vi "GUI_HTT_Logger.vi"() -> ()   [LabVIEW 2013]
uses:
  Shared/GUI_Template/GUI_master/tcp_new_data_event.ctl
  Shared/GUI_Template/GUI_master/tcp new data cluster.ctl
panel:
  out "PellicleMeter 10h":cluster{"Y":dbl[], "Y":dbl[]}[](graph)
  out "PellicleMeter":cluster{"Y":dbl[], "Y":dbl[]}[](graph)
  in  "AI_mean.Channel 0::4":dbl caption="Temperature" min=0.0 max=0.0
  in  "GUIdevice 4":string="HTT-PellicleMeter"
  in  "Energy.Channel 1::2":dbl caption="Energy" min=0.0 max=0.0
  in  "Energy.Channel 0::2":dbl min=0.0 max=20.0
  out "Energy 2 10h":cluster{"Y":dbl[], "Y":dbl[]}[](graph)
  out "Temp Gaia 10h":cluster{"Y":dbl[], "Y":dbl[]}[](graph)
  out "Temp Amps 10h":cluster{"Y":dbl[], "Y":dbl[]}[](graph)
  out "Temp Amps":cluster{"Y":dbl[], "Y":dbl[]}[](graph)
  in  "GUIdevice 3":string="HTT-Temp-Amps"
  in  "Temperature::3":dbl caption="Temperature" min=0.0 max=500.0
  in  "Temperature::1":dbl caption="Temperature" min=0.0 max=500.0
  in  "GUIdevice 2":string="HTT-Pulsar"
  in  "Wavelength.Channel1::2":string(combo)="800"
  in  "EnergyRange.Channel1::2":string(combo)="4.00J"
  in  "MeasurementMode.Channel1::2":string(combo)="Energy"
  in  "Wavelength.Channel0::2":string(combo)="800"
  in  "EnergyRange.Channel0::2":string(combo)="4.00J"
  in  "MeasurementMode.Channel0::2":string(combo)="Energy"
  out "tcp data event":T1
  out "error IO 2":errorcluster
  in  "ExternalTrigger.Channel1::2":bool=TRUE caption="Blank Button"
  in  "GUIdevice 1":string="HTT-Temp-Gaia"
  in  "?":bool
  out "Energy 2":cluster{"Y":dbl[], "Y":dbl[]}[](graph)
  out "Temp Gaia":cluster{"Y":dbl[], "Y":dbl[]}[](graph)
  out "Energy 1":cluster{"Y":dbl[], "Y":dbl[]}[](graph)
  out "Energy 1 10h":cluster{"Y":dbl[], "Y":dbl[]}[](graph)
  # "Please re-enter these values after starting the program or restarting the device!"
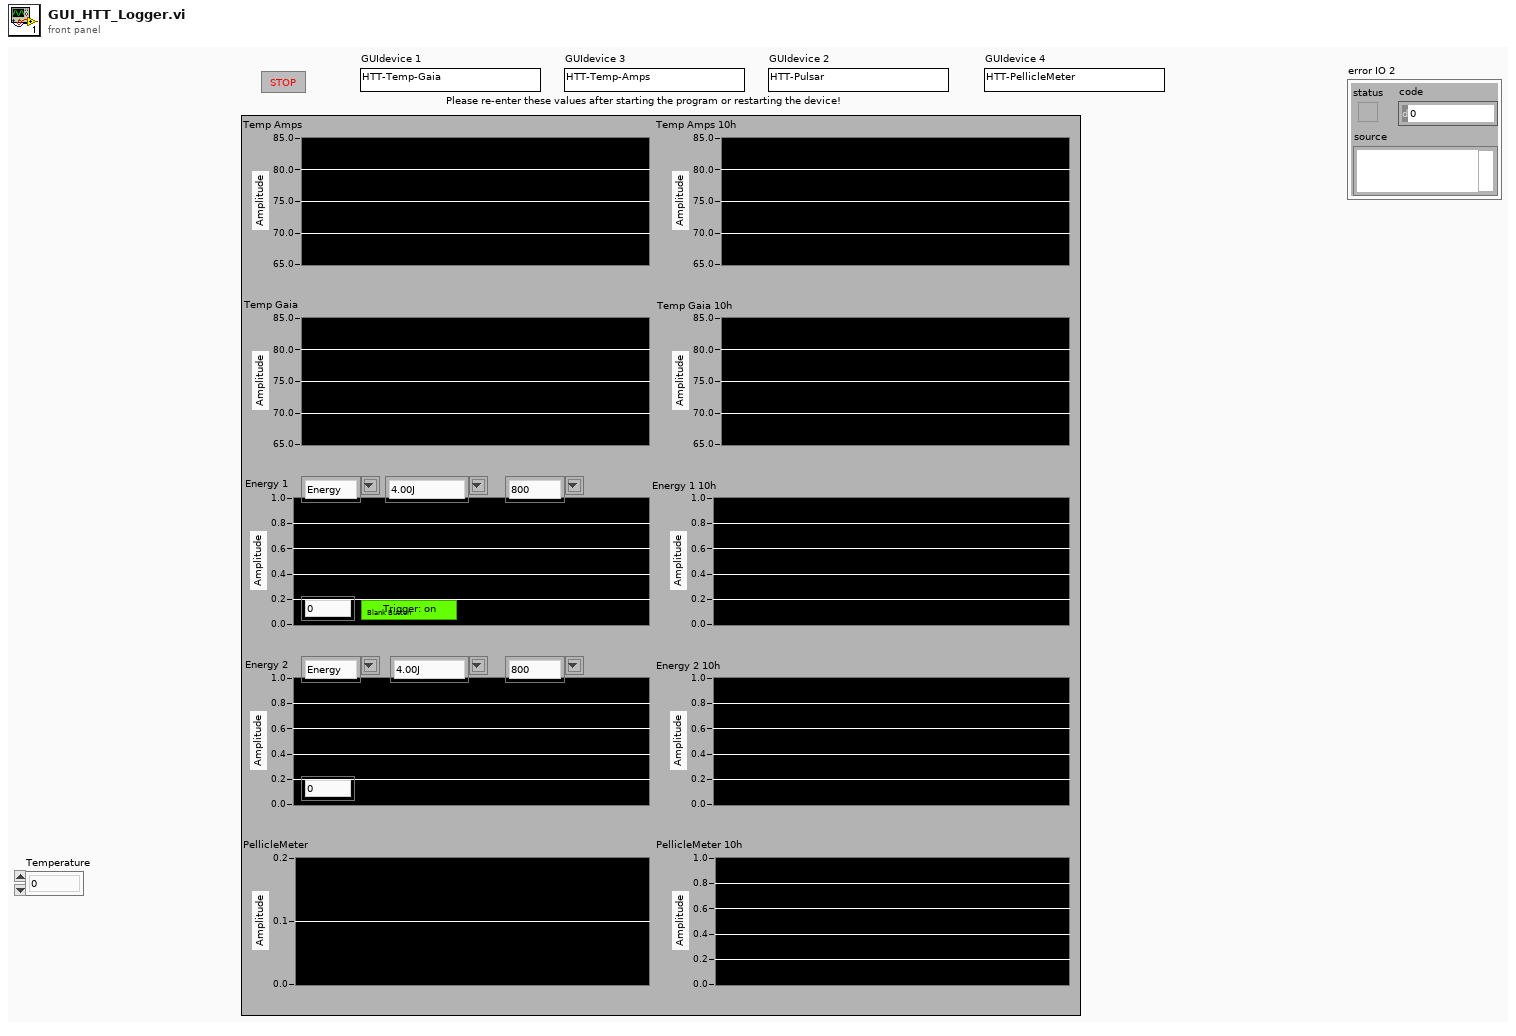
[diagram p1: front panel]
types:
  T1 = typedef "tcp_new_data_event.ctl" = refnum<user-event>
  T2 = enum16{"open", "replace", "create", "open or create", "replace or create", "replace or create with confirmation"}
  T3 = typedef "tcp new data cluster.ctl" = cluster{"EventEnum":enum16{"new data", "connection status update"}, "Device name":string}
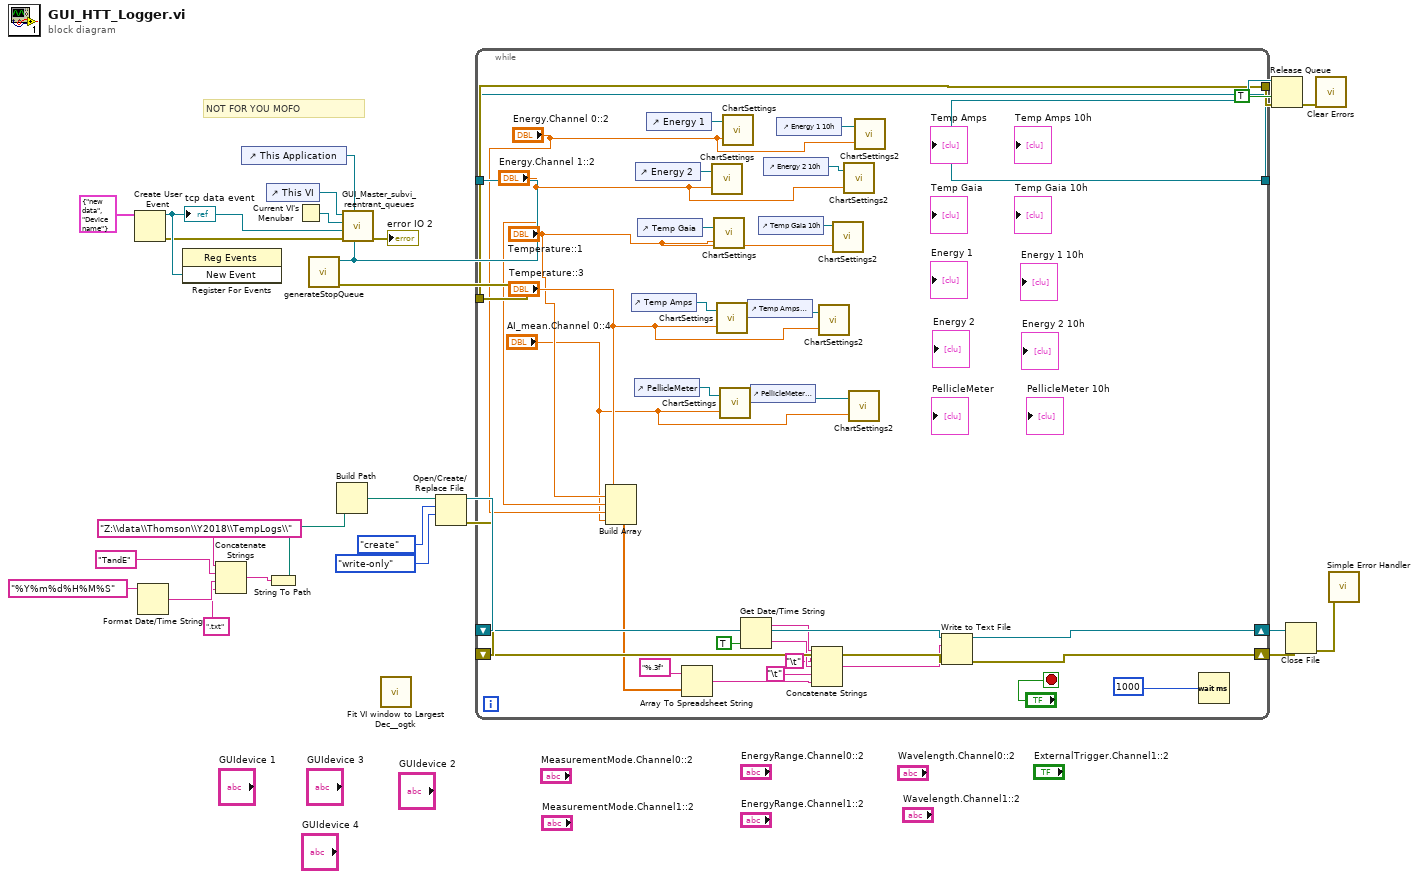
[diagram p0: block diagram]
diagram:
  # "NOT FOR YOU MOFO"
  n1 = Create User Event(user event datatype=T3 {"EventEnum"=enum."new data", "Device name"="Device name"} ("New Event")) -> (user event=w23:refnum<user-event>, error out=w22:errorcluster)  [unwired: 1 in]
  "tcp data event" <- w23
  n2 = Format Date/Time String(time format string (%c)="%Y%m%d%H%M%S") -> (date/time string=w3:string)  [unwired: 2 in]
  n3 = register-events(w23) -> ()  [unwired: 2 in, 2 out]
  n4 = Concatenate Strings("Z:\\data\\Thomson\\Y2018\\TempLogs\\", "TandE", w3, ".txt" ("string")) -> (w5:string)
  n5 = control-ref of="This Application"() -> (w24:refnum<vi>)
  n6 = control-ref of="This VI"() -> (w19:refnum<vi>)
  n7 = String To Path(string=w5) -> (path=w4:path)
  n8 = Current VI's Menubar() -> (w20:refnum<k9>)
  n9 = call "generateStopQueue.vi"() -> ("error out"=w17:errorcluster, "STOP Queue out"=w16:refnum<queue>)  [unwired: 10 in]
  n10 = Build Path(name or relative path=w4) -> (appended path=w8:path)  [unwired: 1 in]
  n11 = call "GUI_Master_subvi_reentrant_queues.vi"("STOP Queue in"=w16, "This Application"=w24, "error in (no error)"=w22, "tcp data event"=w23, "Caller menu reference"=w20, "Caller VI ref"=w19) -> ("error out"=→"error IO 2":errorcluster)  [unwired: 5 in]
  n12 = call <userlib>:"Fit VI window to Largest Dec__ogtk.vi"() -> ()  [unwired: 6 in, 2 out]
  n13 = Open/Create/Replace File(file path (use dialog)=w8, operation (0:open)=T2."create", access (0:read/write)=enum16{"read/write", "read-only", "write-only"}."write-only") -> (refnum out=w13:refnum<file>, error out=w10:errorcluster)  [unwired: 1 in, 3 out]
  n14 = while {
    tunnel: [w59] -> w26
    tunnel: w17 -> [w59]
    tunnel: w16 -> [w58]
    tunnel: [w58] -> w25
    shift-right: [w56] -> w11
    shift-left: w13 -> [w57]
    shift-right: [w54] -> w9
    shift-left: w10 -> [w55]
    stop <- "?" stop-if-true
    n15 = Build Array("Temperature::3", "Temperature::1", "Energy.Channel 1::2", "Energy.Channel 0::2", "AI_mean.Channel 0::4") -> (w52:dbl[])
    n16 = control-ref of="Temp Amps"() -> (w43:refnum<vi>)
    n17 = control-ref of="PellicleMeter"() -> (w31:refnum<vi>)
    n18 = control-ref of="Energy 2"() -> (w41:refnum<vi>)
    n19 = control-ref of="Temp Gaia"() -> (w42:refnum<vi>)
    n20 = control-ref of="Energy 1"() -> (w40:refnum<vi>)
    n21 = Array To Spreadsheet String(array=w52, 3:"%.3f" ("format string")) -> (spreadsheet string=w45:string)  [unwired: 1 out]
    n22 = call "ChartSettings.vi"("Numeric"="Energy.Channel 1::2", "XY Graph Ref in"=w41) -> ()  [unwired: 1 in]
    n23 = call "ChartSettings.vi"("Numeric"="Temperature::1", "XY Graph Ref in"=w42) -> ()  [unwired: 1 in]
    n24 = call "ChartSettings.vi"("Numeric"="Temperature::3", "XY Graph Ref in"=w43) -> ()  [unwired: 1 in]
    n25 = call "ChartSettings.vi"("Numeric"="AI_mean.Channel 0::4", "XY Graph Ref in"=w31) -> ()  [unwired: 1 in]
    n26 = call "ChartSettings.vi"("Numeric"="Energy.Channel 0::2", "XY Graph Ref in"=w40) -> ()  [unwired: 1 in]
    n27 = Get Date/Time String(want seconds? (F)=TRUE) -> (date string=w50:string, time string=w49:string)  [unwired: 2 out]
    n28 = control-ref of="Temp Amps 10h"() -> (w39:refnum<vi>)
    n29 = control-ref of="PellicleMeter 10h"() -> (w30:refnum<vi>)
    n30 = control-ref of="Temp Gaia 10h"() -> (w37:refnum<vi>)
    n31 = control-ref of="Energy 2 10h"() -> (w33:refnum<vi>)
    n32 = control-ref of="Energy 1 10h"() -> (w35:refnum<vi>)
    n33 = Concatenate Strings(w50, "\t" ("Tab"), w49, "\t" ("Tab"), w45) -> (w44:string)
    n34 = call "ChartSettings2.vi"("Numeric"="Temperature::3", "XY Graph Ref in"=w39) -> ()  [unwired: 1 in]
    n35 = call "ChartSettings2.vi"("Numeric"="Temperature::1", "XY Graph Ref in"=w37) -> ()  [unwired: 1 in]
    n36 = call "ChartSettings2.vi"("Numeric"="Energy.Channel 1::2", "XY Graph Ref in"=w33) -> ()  [unwired: 1 in]
    n37 = call "ChartSettings2.vi"("Numeric"="AI_mean.Channel 0::4", "XY Graph Ref in"=w30) -> ()  [unwired: 1 in]
    n38 = call "ChartSettings2.vi"("Numeric"="Energy.Channel 0::2", "XY Graph Ref in"=w35) -> ()  [unwired: 1 in]
    n39 = Write to Text File(file (use dialog)=w57, text=w44, error in=w55) -> (refnum out=w56:refnum<file>, error out=w54:errorcluster)  [unwired: 1 in, 1 out]
    n40 = Wait (ms)(milliseconds to wait=u32 1000) -> ()  [unwired: 1 out]
  }
  n41 = Release Queue(queue=w25, force destroy? (F)=TRUE, error in (no error)=w26) -> (error out=w28:errorcluster)  [unwired: 2 out]
  n42 = Close File(refnum=w11, error in=w9) -> (error out=w12:errorcluster)  [unwired: 1 out]
  n43 = call <vilib>:"Clear Errors.vi"("error in (no error)"=w28) -> ()  [unwired: 6 in, 1 out]
  n44 = call <vilib>:"Simple Error Handler.vi"("error in (no error)"=w12) -> ()  [unwired: 1 in, 8 out]
